vi "HP1200_330_get_TempPmpBot.vi"(7 "device_addr":u16=22, 8 "error in":errorcluster, 11 "conn_id_in":refnum<k5>) -> (0 "error out":errorcluster, 1 "response":string, 2 "temp":i16, 3 "conn_id_out":refnum<k5>, 4 "status":bool)   [LabVIEW 2019]
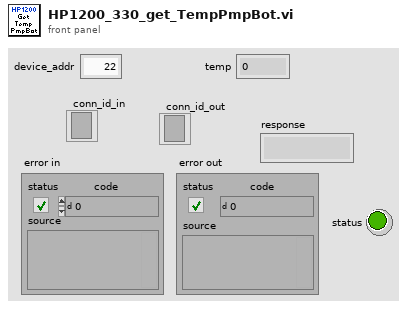
[diagram p1: front panel]
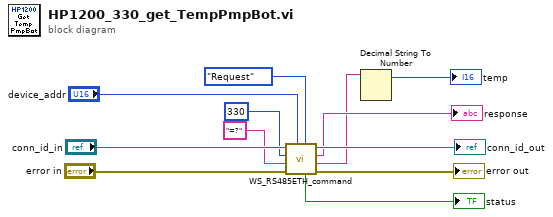
[diagram p0: block diagram]
diagram:
  n1 = call "WS_RS485ETH_command.vi"("action"=enum16{"Request", "Control"}."Request", "device_addr"="device_addr", "error in"="error in", "data_string"="=?" ("data"), "param_num"=u16 330, "conn_id_in"="conn_id_in") -> ("error out"=→"error out":errorcluster, "data_out"=w1:string, "response"=→"response":string, "conn_id_out"=→"conn_id_out":refnum<k5>, "status"=→"status":bool)  [unwired: 1 in]
  n2 = Decimal String To Number(string=w1) -> (offset past number=→"temp":i32)  [unwired: 2 in, 1 out]
